vi "Drag & Drop End.vi"   [LabVIEW 2015]
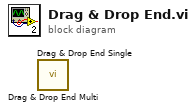
[diagram p0: block diagram]
diagram:
  n1 = call "Drag & Drop End Multi.vi"() -> ()  [unwired: 11 in, 1 out]
  n2 = call "Drag & Drop End Single.vi"() -> ()  [unwired: 11 in, 1 out]
